vi "ROITransform.vi"() -> ()   [LabVIEW 2016]
doc: "This example shows how to compute the histogram of an image or a region in the image. This example also shows how to set up and use the display tools to select and work on different regions in the image interactively."
uses:
  <vilib>/vision/NI_Vision_Development_Module.lvlib
panel:
  out "Image":T1(plugin-control)
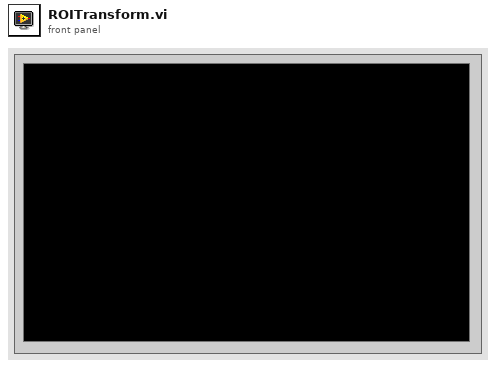
[diagram p1: front panel]
types:
  T1 = typedef "IMAQ Image.ctl" = refnum<image>
  T2 = typedef "IMAQ Line" = cluster{"Start X":i32, "Start Y":i32, "End X":i32, "End Y":i32}
  T3 = cluster{"Origin":cluster{"X":sgl, "Y":sgl}, "Angle (deg)":sgl, "Axis Reference":u32}
  T4 = typedef "ROI Descriptor" = cluster{"Global Rectangle":i32[], "Contours":cluster{"ID":enum32{"External", "Internal"}, "Type":u32, "Coordinates":i32[]}[]}
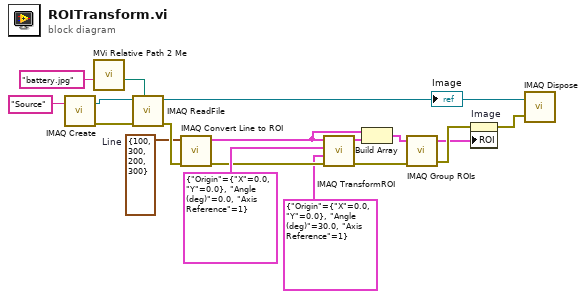
[diagram p0: block diagram]
diagram:
  w3 = T2 {"Start X"=100, "Start Y"=300, "End X"=200, "End Y"=300}  # Line
  n1 = call "IMAQ Create"("Image Name"="Source") -> ("New Image"=w18:T1, "error out"=w17:errorcluster)  [unwired: 4 in]
  n2 = call "MVi Relative Path 2 Me.vi"("Relative Path"="battery.jpg") -> ("Appended Dir"=w1:path)  [unwired: 5 in, 1 out]
  n3 = call "IMAQ ReadFile"("File Path"=w1, "error in (no error)"=w17, "Image"=w18) -> ("error out"=w15:errorcluster, "Image Out"=w12:T1)  [unwired: 4 in, 3 out]
  "Image" <- w12
  n4 = call "IMAQ Convert Line to ROI"("error in (no error)"=w15, "Line"=w3) -> ("error out"=w13:errorcluster, "ROI Descriptor"=w9:T4)  [unwired: 7 in]
  n5 = call "IMAQ TransformROI"("error in (no error)"=w13, "New Reference"=T3 {"Origin"={"X"=0.0, "Y"=0.0}, "Angle (deg)"=30.0, "Axis Reference"=1} ("Base Reference"), "Base Reference"=T3 {"Origin"={"X"=0.0, "Y"=0.0}, "Angle (deg)"=0.0, "Axis Reference"=1}, "ROI Descriptor"=w9) -> ("error out"=w7:errorcluster, "ROI Descriptor out"=w8:T4)  [unwired: 6 in]
  n6 = Build Array(w9, w8) -> (w6:T4[])
  n7 = call "IMAQ Group ROIs"("error in (no error)"=w7, "ROI Descriptors"=w6) -> ("error out"=w5:errorcluster, "ROI Descriptor out"=w4:T4)  [unwired: 2 in]
  n8 = property on="Image" class="ImageControl"(error in=w5, "ROI"=w4) -> (error out=w11:errorcluster)  [unwired: 1 in, 1 out]
  n9 = call "IMAQ Dispose"("Image"=w12, "error in (no error)"=w11) -> ()  [unwired: 4 in, 1 out]
